vi "IPSHTBoxRead.vi"(8 "error in (no error)":errorcluster, 11 "IP in":string="192.168.1.23") -> (0 "RH2D":dbl[][](array[numeric]), 1 "Temp2D":dbl[][](array[numeric]), 2 "cluster":T1(array[cluster]), 3 "IP out":string="192.168.1.23", 4 "SHTListName":string[](array[string]), 5 "status":bool, 6 "error out":errorcluster)   [LabVIEW 2019]
uses:
  <vilib>/httpClient/LabVIEWHTTPClient.lvlib
panel:
  out "body":string
  out "headers":string
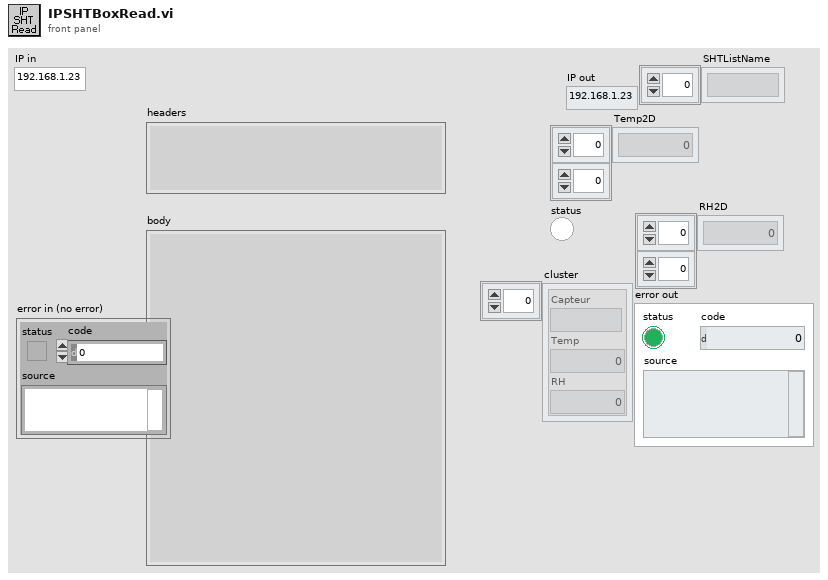
[diagram p1: front panel]
types:
  T1 = cluster{"Capteur":string, "Temp":dbl, "RH":dbl}[]
  T2 = cluster{"status":bool, "code":bool, "source":bool}
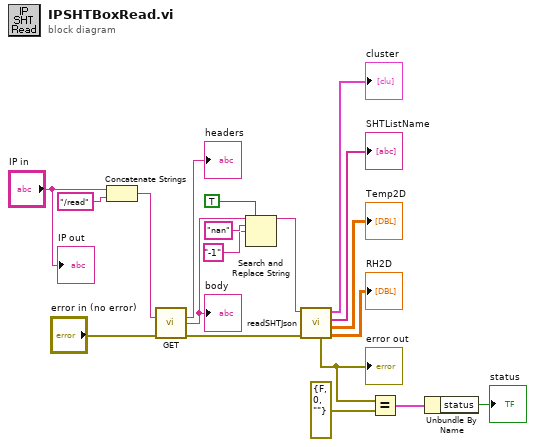
[diagram p0: block diagram]
diagram:
  n1 = Concatenate Strings("IP in", "/read" ("address")) -> (w16:string)
  n2 = call <vilib>:"GET.vi"("url"=w16, "error in (no error)"="error in (no error)") -> ("headers"=→"headers":string, "body"=w9:string, "error out"=w10:errorcluster)  [unwired: 10 in, 1 out]
  "body" <- w9
  n3 = Search and Replace String(replace all?=TRUE ("replace all? (F)"), input string=w9, search string="nan", replace string="-1" ("replace string (\"\")")) -> (result string=w5:string)  [unwired: 4 in, 3 out]
  n4 = call "readSHTJson.vi"("JSON in"=w5, "error in (no error)"=w10) -> ("error out"=w4:errorcluster, "cluster"=→"cluster":T1, "SHTListName"=→"SHTListName":string[], "Temp2D"=→"Temp2D":dbl[][], "RH2D"=→"RH2D":dbl[][])  [unwired: 4 in]
  "error out" <- w4
  n5 = Equal?(x=w4, y=errorcluster {"status"=FALSE, "code"=0, "source"=""}) -> (x = y?=w2:T2)
  n6 = Unbundle By Name(w2) -> ("status"=→"status":bool)
  "IP out" <- "IP in"
